vi "Initialize Active Options.vi"(8 "error in (no error)":errorcluster, 11 "Active Option View Definition in":refnum<class "Active Option View Definition.lvclass">) -> (0 "error out":errorcluster, 3 "Active Option View Definition out":refnum<class "Active Option View Definition.lvclass">)   [LabVIEW 2019, in "Active Option View Definition.lvclass"]
uses:
  <vilib>/gpm_packages/@cs/Car-wash/Source/Active Station View Definition/Active Station View Definition/Active Option View Definition.lvclass
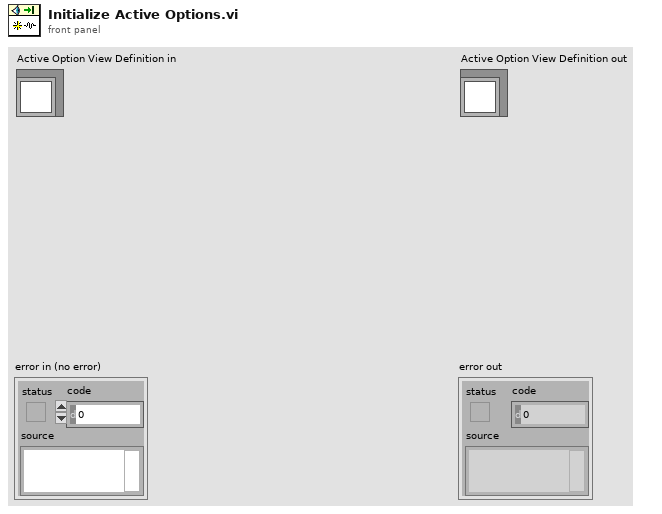
[diagram p1: front panel]
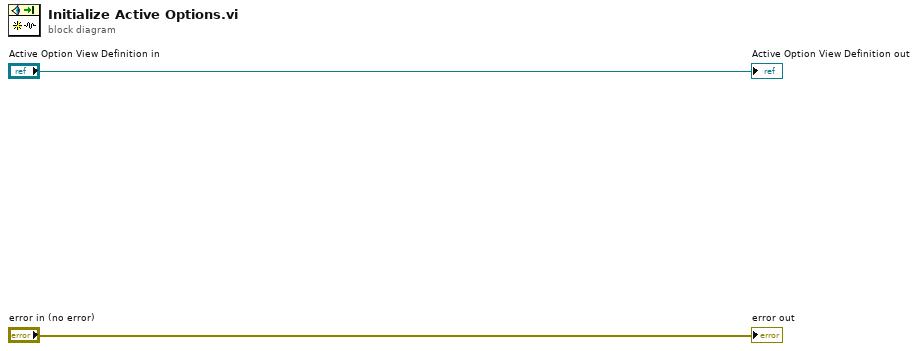
[diagram p0: block diagram]
diagram:
  "error out" <- "error in (no error)"
  "Active Option View Definition out" <- "Active Option View Definition in"
